vi "X Units.vi"(1 "Interval Units (points)":enum16{"Points", "Data"}(ring), 2 "Interval (h)":dbl, 3 "X-array":dbl[](array[numeric])) -> (0 "h (points)":i32)   [LabVIEW 2016, in "xy_utilities.lvlib"]
doc: "Calculate <b>h</b> in appropriate units."
uses:
  xy_utilities.lvlib
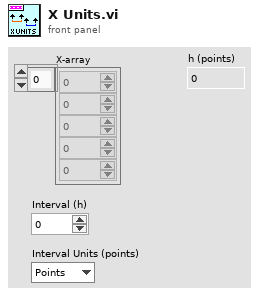
[diagram p1: front panel]
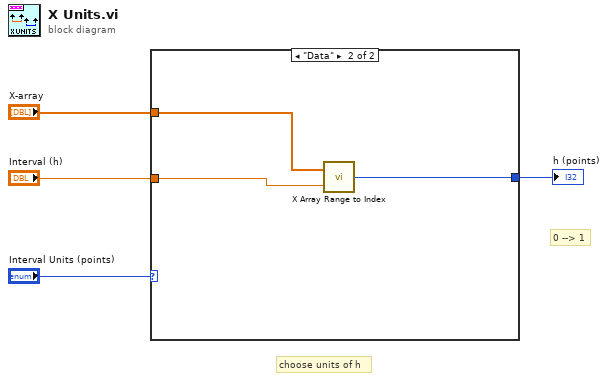
[diagram p0: block diagram]
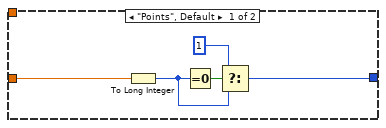
[diagram p2: hidden frame]
diagram:
  # "0 --> 1"
  # "choose units of h"
  n1 = case shown="\"Data\"" "Interval Units (points)" {
    tunnel: "Interval (h)" -> [w9 w12]
    tunnel: [w5 w11] -> w1
    tunnel: "X-array" -> [_ w10]
    frame "Points", Default {
      n2 = To Long Integer(number=w9) -> (32bit integer=w6:i32)
      n3 = Equal To 0?(x=w6) -> (x = 0?=w8:bool)
      n4 = Select(t=1, s=w8, f=w6) -> (s? t:f=w5:i32)
    }
    frame "Data" {
      n5 = call "X Array Range to Index.vi"("X Range (data)"=w12, "X-array"=w10) -> ("X Range (points)"=w11:i32)
    }
  }
  "h (points)" <- w1
